vi "System-AsyncUserVI.vi"(11 "DSI Reference":refnum<class "DCM-DSI.lvclass">) -> ()   [LabVIEW 2016, in "DSI-RT.lvlib"]
uses:
  DSI-RT.lvlib
  Classes/DCM-DSI/DCM-DSI.lvclass
  Classes/DCM-DSI/Write dt.vi
  Classes/DCM-DSI/Write LoopCount.vi
  <vilib>/addons/Software Calibration Management/xSCM/CalPoint.xnode
  <vilib>/addons/Software Calibration Management/xSCM/FaultPoint.xnode
  <vilib>/addons/Software Calibration Management/xSCM/ni_scm.dll
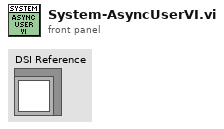
[diagram p1: front panel]
types:
  T1 = typedef "DCM-DSI.lvclass/UserParameter.ctl" = cluster{"Name":string, "Value":dbl}
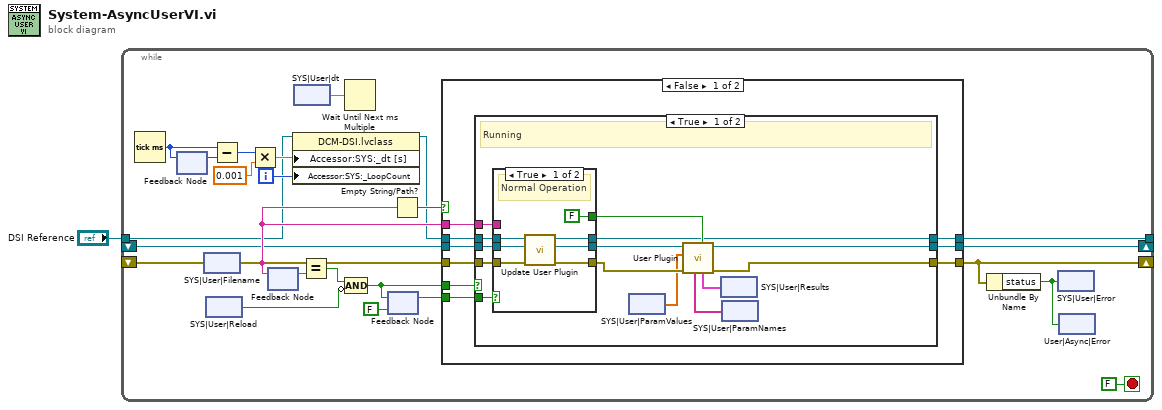
[diagram p0: block diagram]
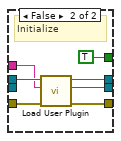
[diagram p2: hidden frame]
diagram:
  n1 = while {
    shift-right: [w13] -> _
    shift-left: _ -> [w25]
    tunnel: "DSI Reference" -> [w4]
    shift-right: [w12] -> _
    shift-left: _ -> [w2]
    tunnel: [w15] -> _
    i -> [w6]
    stop <- FALSE stop-if-true
    n2 = Tick Count (ms)() -> (millisecond timer value=w11:u32)
    n3 = feedback #1() -> (w8:u32)  [unwired: 1 in]
    n4 = feedback-in #1(w11) -> ()
    n5 = xnode "SYS|User|Filename"() -> ("Value"=w18:string)
    n6 = xnode "SYS|User|Reload"() -> ("Value"=w23:bool)
    n7 = Subtract(x=w11, y=w8) -> (x-y=w9:u32)
    n8 = Multiply(x=w9, y=0.001) -> (x*y=w7:sgl)
    n9 = feedback #2() -> (w20:string)  [unwired: 1 in]
    n10 = feedback-in #2(w18) -> ()
    n11 = property class="DCM-DSI.lvclass"(reference=w4, "Accessor:SYS:_dt [s]"=w7, "Accessor:SYS:_LoopCount"=w6) -> (reference out=w3:refnum<class "DCM-DSI.lvclass">)  [unwired: 1 in, 1 out]
    n12 = xnode "SYS|User|dt"() -> ("Value"=w5:sgl)
    n13 = Equal?(x=w18, y=w20) -> (x = y?=w21:bool)
    n14 = Wait Until Next ms Multiple(millisecond multiple=w5) -> ()  [unwired: 1 out]
    n15 = Compound Arithmetic op=AND(w21, invert w23) -> (w17:bool)
    n16 = feedback #3(FALSE) -> (w16:bool)
    n17 = feedback-in #3(w17) -> ()
    n18 = Empty String/Path?(string/path=w18) -> (empty?=w19:bool)
    n19 = case shown="False" w19 {
      tunnel: [w72 w125] -> w15
      tunnel: [w71 _] -> w13
      tunnel: w16 -> [w70 _]
      tunnel: w17 -> [w69 _]
      tunnel: w18 -> [w68 _]
      tunnel: w3 -> [w67 w125]
      tunnel: w25 -> [w66 _]
      tunnel: [w65 _] -> w12
      tunnel: w2 -> [w64 _]
      frame False {
        n20 = case shown="True" w69 {
          tunnel: [w76 w124] -> w72
          tunnel: [w73 _] -> w71
          tunnel: w70 -> [w86 _]
          tunnel: w68 -> [w85 _]
          tunnel: w67 -> [w84 w124]
          tunnel: w66 -> [w83 _]
          tunnel: [w75 _] -> w65
          tunnel: w64 -> [w74 _]
          frame True {
            # "Running"
            n21 = case shown="True" w86 {
              tunnel: [w109 w115] -> w82
              tunnel: [w105 w116] -> w81
              tunnel: w85 -> [_ w112]
              tunnel: w84 -> [w108 w117]
              tunnel: w83 -> [w106 w113]
              tunnel: [FALSE ("Initialize") TRUE ("Initialize")] -> w77
              tunnel: [w107 w114] -> w76
              tunnel: w74 -> [w110 _]
              frame True {
                # "Normal Operation"
                n22 = call "Update User Plugin.vi"("error in (no error)"=w106, "Plugin Reference"=w110, "DSI Reference"=w108) -> ("error out"=w105:errorcluster, "Plugin Reference"=w109:refnum<class "DCM-DSI.lvclass">, "DSI Reference"=w107:refnum<class "DCM-DSI.lvclass">)  [unwired: 6 in]
              }
              frame False {
                # "Initialize"
                n23 = call "Load User Plugin.vi"("error in (no error)"=w113, "Name or relative path"=w112, "DSI Reference"=w117) -> ("error out"=w116:errorcluster, "Plugin Reference"=w115:refnum<class "DCM-DSI.lvclass">, "DSI Reference"=w114:refnum<class "DCM-DSI.lvclass">)  [unwired: 6 in]
              }
            }
            n24 = xnode "SYS|User|ParamValues"() -> ("Value"=w78:sgl[])
            n25 = call-dynamic "User Plugin.vi"("Initialize"=w77, "error in (no error)"=w81, "ParamValues"=w78, "DSI Reference"=w82) -> ("error out"=w73:errorcluster, "DSI Reference"=w75:refnum<class "DCM-DSI.lvclass">, "Results"=w79:T1[], "ParamNames"=w80:string[])  [unwired: 4 in]
            n26 = xnode "SYS|User|Results"("Value"=w79) -> ()
            n27 = xnode "SYS|User|ParamNames"("Value"=w80) -> ()
          }
          frame False {
            # "Off"
          }
        }
      }
      frame True {
      }
    }
    n28 = Unbundle By Name(w13) -> ("status"=w14:bool)
    n29 = xnode "SYS|User|Error"("Value"=w14) -> ()
    n30 = xnode "User|Async|Error"("Fault"=w14) -> ()
  }
